vi "TCIPSendCmd.vi"(6 "error in (no error)":errorcluster, 8 "bytes to read":i32=3, 9 "Command":string="*W012003E8", 10 "Port Number":u16=1000, 11 "IP Address":string="192.168.12.200") -> (3 "Output Reading":string, 4 "error out":errorcluster)   [LabVIEW 2013, in "ovenCtrl.lvlib"]
uses:
  ovenCtrl.lvlib
panel:
  # "Inputs"
  # "Outputs"
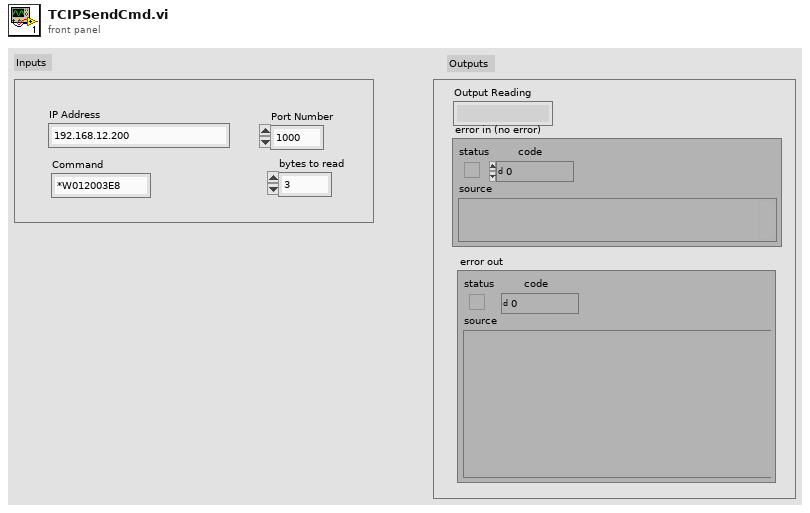
[diagram p1: front panel]
types:
  T1 = enum16{"Standard", "Buffered", "CRLF", "Immediate"}
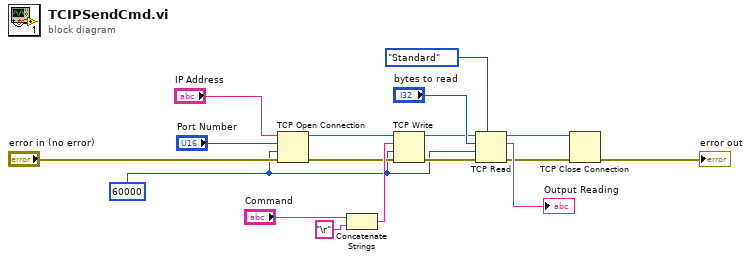
[diagram p0: block diagram]
diagram:
  w1 = 60000 ("timeout ms (60000)")
  n1 = TCP Open Connection(address="IP Address", remote port or service name="Port Number", timeout ms (60000)=w1, error in (no error)="error in (no error)") -> (connection ID=w11:refnum<k5>, error out=w6:errorcluster)  [unwired: 1 in]
  n2 = Concatenate Strings("Command", "\r") -> (w16:string)
  n3 = TCP Write(connection ID=w11, data in=w16, error in (no error)=w6, 9:w1) -> (connection ID out=w8:refnum<k5>, error out=w5:errorcluster)  [unwired: 1 out]
  n4 = TCP Read(connection ID=w8, bytes to read="bytes to read", error in (no error)=w5, 7:T1."Standard" ("mode (standard)"), 9:w1) -> (connection ID out=w14:refnum<k5>, data out=→"Output Reading":string, error out=w4:errorcluster)
  n5 = TCP Close Connection(connection ID=w14, error in (no error)=w4) -> (error out=→"error out":errorcluster)  [unwired: 1 in, 1 out]
